vi "Continue.vi"() -> ()   [LabVIEW 2017]
panel:
  in  "Delay (ms)":u32=1000
  out "Continue":bool
  in  "Yes":bool
  in  "stop":bool
  in  "No of Sweeps":i32=1
  out "Sweep":i32
  out "Graph":cluster{"Y":dbl[], "Y":dbl[]}[](graph)
  in  "Number of Points":i32=50 min=10 max=10000 step=1
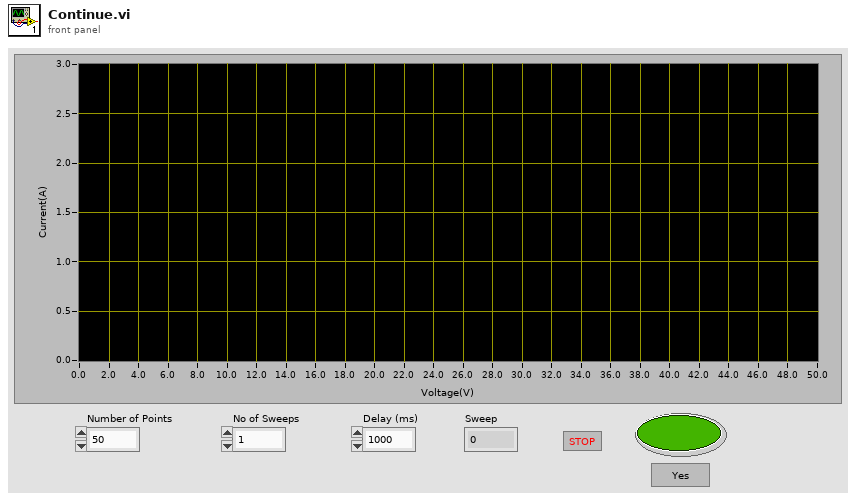
[diagram p1: front panel]
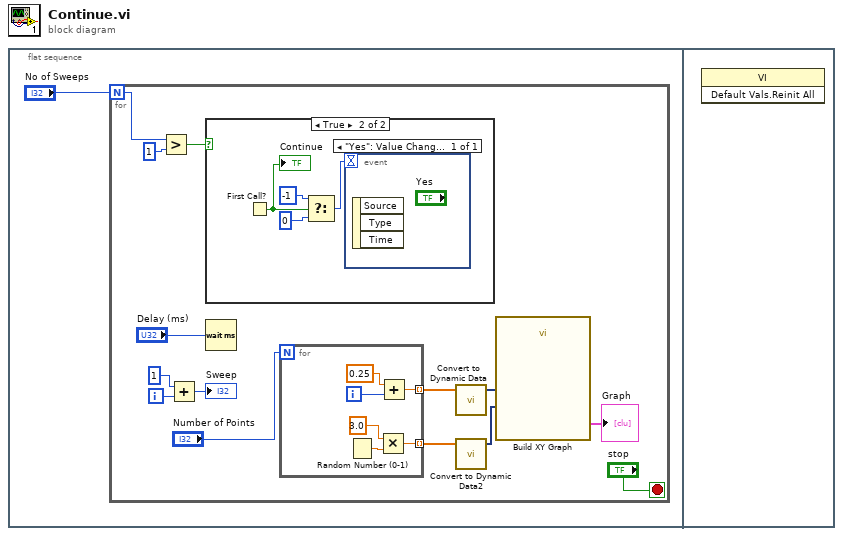
[diagram p0: block diagram]
diagram:
  n1 = flat-sequence {
    frame #0 {
      n2 = for {
        N: "No of Sweeps" -> [w3]
        i -> [w9]
        stop <- "stop" stop-if-true
        n3 = Greater?(x=w3, y=1) -> (0:w5:bool)
        n4 = Add(x=1, y=w9) -> (x+y=→"Sweep":i32)
        n5 = case shown="True" w5 {
          frame False {
          }
          frame True {
            n6 = First Call?() -> (First Call?: T/F=w16:bool)
            "Continue" <- w16
            n7 = Select(t=-1, s=w16, f=0) -> (s? t:f=w19:i32)
            n8 = event shown="[0] \"Yes\": Value Change;  Timeout" {
              selector: _ -> [_]
              dyn-events: _ -> [_]
              timeout: w19 -> [_]
              event "Yes": Value Change; Timeout {
                n9 = event-data() -> ()  [unwired: 1 in, 3 out]
              }
            }
          }
        }
        n10 = Wait (ms)(milliseconds to wait="Delay (ms)") -> ()  [unwired: 1 out]
        n11 = for {
          N: "Number of Points" -> [_]
          tunnel: [w21] -> w10 mode=indexing
          tunnel: [w20] -> w11 mode=indexing
          i -> [w22]
          n12 = Random Number (0-1)() -> (number: 0 to 1=w23:dbl)
          n13 = Multiply(x=3.0, y=w23) -> (x*y=w20:dbl)
          n14 = Add(x=0.25 ("y"), y=w22) -> (x+y=w21:dbl)
        }
        n15 = call "Convert to Dynamic Data"("Array"=w10) -> ("Dynamic Data Type"=w15:dynamicdata)  [unwired: 3 in]
        n16 = call "Convert to Dynamic Data2"("Array"=w11) -> ("Dynamic Data Type"=w14:dynamicdata)  [unwired: 3 in]
        n17 = call "Build XY Graph"("Y Input"=w14, "X Input"=w15) -> ("XY Graph"=→"Graph":cluster{"X":dbl[], "Y":dbl[]}[])  [unwired: 8 in, 1 out]
      }
    }
    frame #1 {
      n18 = invoke class="VI" method="Default Vals.Reinit All"() -> ()  [unwired: 3 in, 3 out]
    }
  }
